vi "sketch_test.vi"() -> ()   [LabVIEW 2021]
panel:
  out "Horizon":i16
  out "Verticaly":i16
  in  "Left":bool
  in  "Right":bool
  in  "Down":bool
  in  "UP":bool
  in  "stop":bool
  out "LABVIEW - a - SKETCH":picture
  in  "Boolean":bool
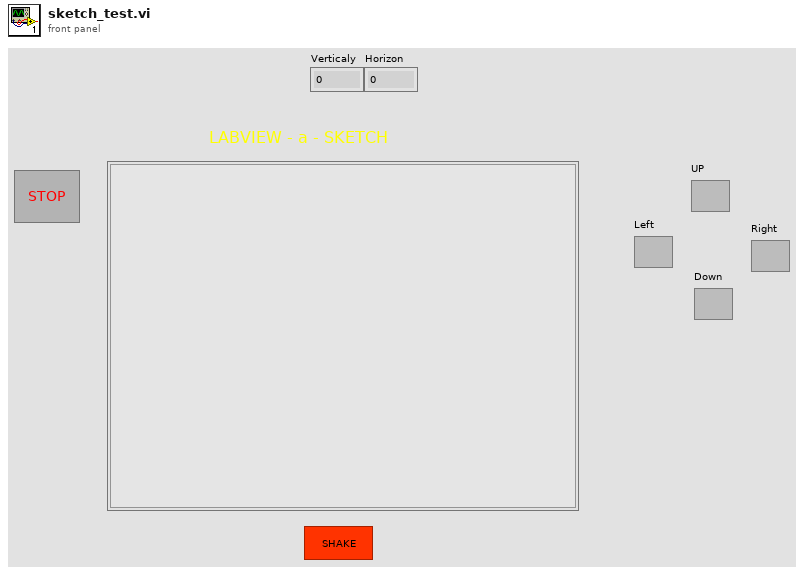
[diagram p1: front panel]
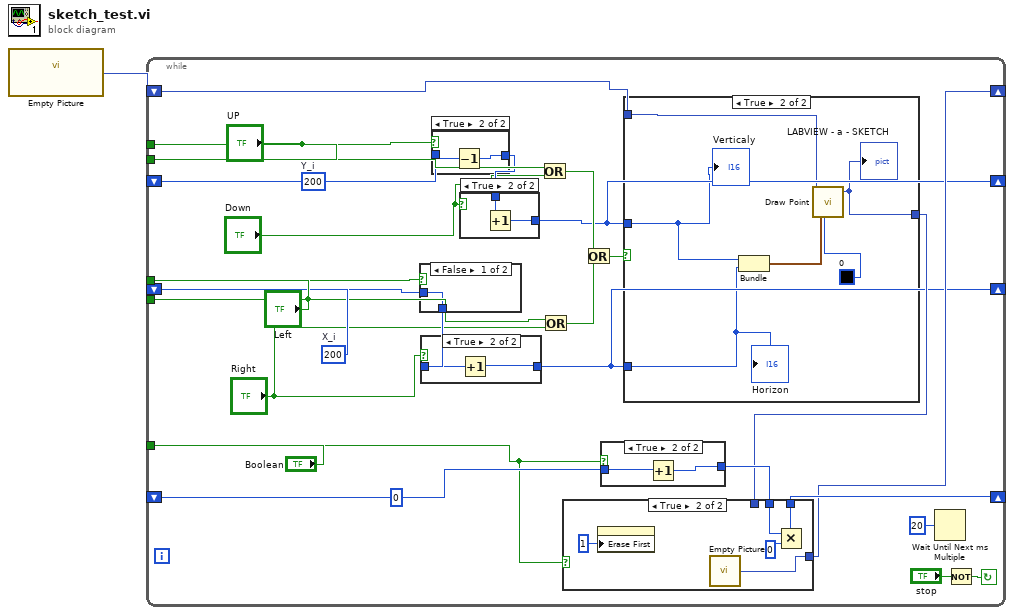
[diagram p0: block diagram]
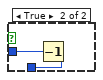
[diagram p6: hidden frame]
diagram:
  w1 = 200  # X_i
  w2 = 200  # Y_i
  n1 = call "Empty Picture"() -> ("empty picture"=w7:picture)
  n2 = while {
    shift-left: 0 -> [w26]
    shift-right: [w24] -> _
    shift-left: w7 -> [w27]
    shift-right: [w22] -> _
    tunnel: "Boolean" -> [w21]
    tunnel: "Left" -> [w19]
    tunnel: "Left" -> [w18]
    tunnel: "UP" -> [w17]
    tunnel: "UP" -> [w16]
    shift-right: [w11] -> _
    shift-left: w2 -> [w15]
    shift-right: [w10] -> _
    shift-left: w1 -> [w13]
    stop <- w31 continue-if-true
    n3 = case shown="False" w19 {
      tunnel: [w53 w55] -> w12
      tunnel: w13 -> [w53 w54]
      frame False {
      }
      frame True {
        n4 = Decrement(x=w54) -> (x-1=w55:i32)
      }
    }
    n5 = case shown="True" "Right" {
      tunnel: [w50 w52] -> w10
      tunnel: w12 -> [w50 w51]
      frame False {
      }
      frame True {
        n6 = Increment(x=w51) -> (x+1=w52:i32)
      }
    }
    n7 = case shown="True" w17 {
      tunnel: [w59 w61] -> w14
      tunnel: w15 -> [w59 w60]
      frame False {
      }
      frame True {
        n8 = Decrement(x=w60) -> (x-1=w61:i32)
      }
    }
    n9 = case shown="True" "Down" {
      tunnel: [w56 w58] -> w11
      tunnel: w14 -> [w56 w57]
      frame False {
      }
      frame True {
        n10 = Increment(x=w57) -> (x+1=w58:i32)
      }
    }
    n11 = Or(x=w16, y="Down") -> (x .or. y?=w29:bool)
    n12 = Or(x=w18, y="Right") -> (x .or. y?=w30:bool)
    n13 = Or(x=w29, y=w30) -> (x .or. y?=w28:bool)
    n14 = case shown="True" w21 {
      tunnel: w26 -> [w33 w35]
      tunnel: [w33 w34] -> w25
      frame False {
      }
      frame True {
        n15 = Increment(x=w35) -> (x+1=w34:i32)
      }
    }
    n16 = case shown="True" w28 {
      tunnel: w27 -> [w43 w48]
      tunnel: [w43 w47] -> w23
      tunnel: w11 -> [_ w46]
      tunnel: w10 -> [_ w45]
      frame False {
      }
      frame True {
        n17 = Bundle("Y_i"=w46, "X_i"=w45) -> (w44:cluster{"Y_i":i32, "X_i":i32})  [unwired: 1 in]
        n18 = call <vilib>:"Draw Point.vi"("picture"=w48, "point(x,y)"=w44, "color(black)"=u32 0 ("PEN COLOR")) -> ("new picture"=w47:picture)  [unwired: 6 in]
        "LABVIEW - a - SKETCH" <- w47
        "Verticaly" <- w46
        "Horizon" <- w45
      }
    }
    n19 = case shown="True" w21 {
      tunnel: w25 -> [w37 w41]
      tunnel: [w37 w40] -> w24
      tunnel: w23 -> [w36 _]
      tunnel: [w36 w39] -> w22
      frame False {
      }
      frame True {
        n20 = property on="LABVIEW - a - SKETCH" class="Pict"("Erase First"=u8 1 ("Write Attribute")) -> ()  [unwired: 2 in, 2 out]
        n21 = call "Empty Picture"() -> ("empty picture"=w39:picture)
        n22 = Multiply(x=w41, y=0) -> (x*y=w40:i32)
      }
    }
    n23 = Wait Until Next ms Multiple(millisecond multiple=u32 20) -> ()  [unwired: 1 out]
    n24 = Not(x="stop") -> (.not. x?=w31:bool)
  }
